vi "Init_S.vi"() -> (1 "All_info":string[][](array[string]), 2 "Title":string, 3 "Path_out":string[](array[string]))   [LabVIEW 2014]
uses:
  <vilib>/Utility/file.llb/Read From Spreadsheet File (string).vi
panel:
  in  "Path":path=path "C:/CS-BarCode/Setting Data/Com.ini"
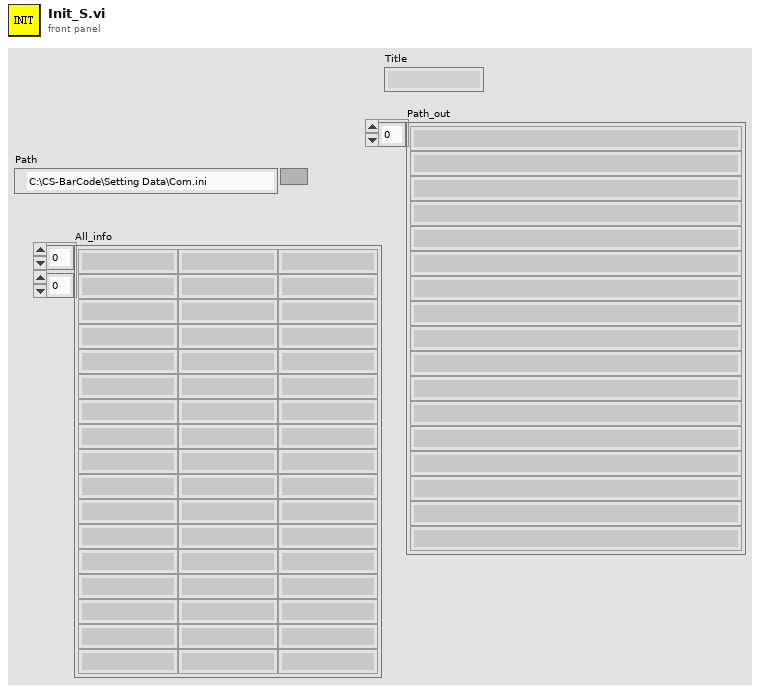
[diagram p1: front panel]
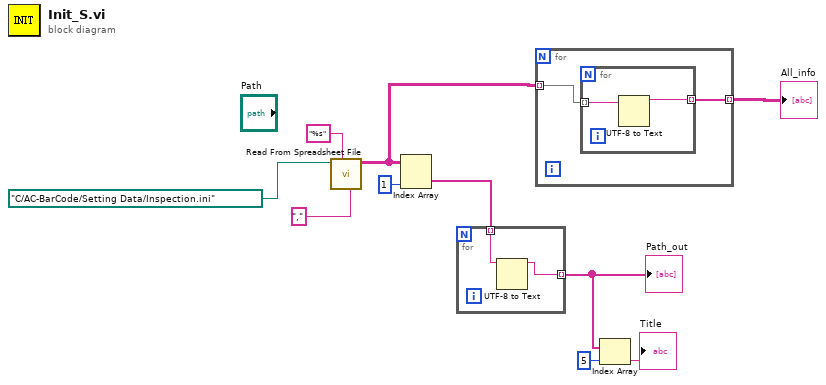
[diagram p0: block diagram]
diagram:
  n1 = call-poly <vilib>:"Read From Spreadsheet File.vi"("delimiter (\\t)"="," ("delimiter (\\t)"), "format (%s)"="%s", "file path (dialog if empty)"=path "C:/AC-BarCode/Setting Data/Inspection.ini") -> ("all rows"=w2:string[][])  [unwired: 4 in, 4 out]
  n2 = Index Array(array=w2, index (col)=1 ("disabled index (col)")) -> (element=w6:string[])  [unwired: 1 in]
  n3 = for {
    tunnel: w6 -> [w12] mode=indexing
    tunnel: [w11] -> w5 mode=indexing
    n4 = UTF-8 to Text(11:w12) -> (3:w11:string)  [unwired: 2 in, 1 out]
  }
  "Path_out" <- w5
  n5 = for {
    tunnel: w2 -> [w14] mode=indexing
    tunnel: [w13] -> w1 mode=indexing
    n6 = for {
      tunnel: w14 -> [w16] mode=indexing
      tunnel: [w15] -> w13 mode=indexing
      n7 = UTF-8 to Text(11:w16) -> (3:w15:string)  [unwired: 2 in, 1 out]
    }
  }
  "All_info" <- w1
  n8 = Index Array(array=w5, index=5) -> (element=→"Title":string)
